vi "ULx Create 1D Waveform (1Samp).vi"(0 "t0":ext format="%#_10g", 5 "dt":dbl, 7 "data Array":dbl[](array[numeric]) format="%0.2f", 9 "channelName Array":string[](array[string]), 11 "error in":errorcluster) -> (4 "data":waveform(dbl)[](array[waveform]), 15 "error out":errorcluster)   [LabVIEW 2020]
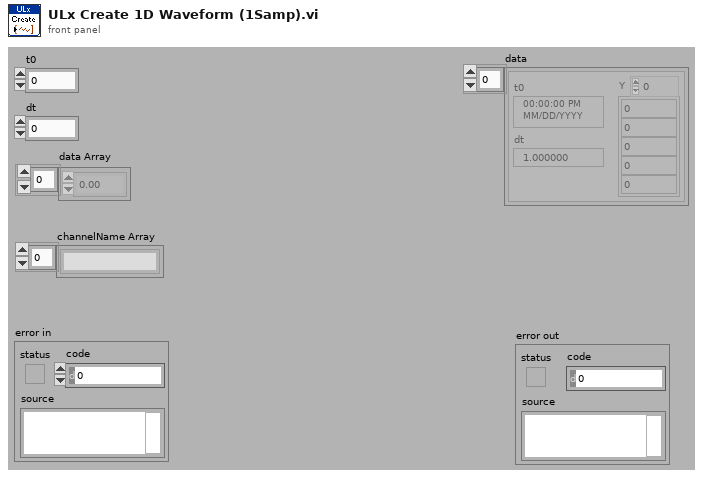
[diagram p1: front panel]
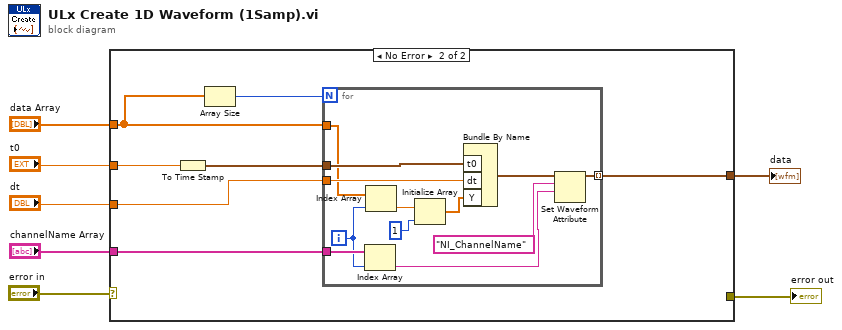
[diagram p0: block diagram]
diagram:
  n1 = case shown="No Error" "error in" {
    selector: "error in" -> [w8 _]
    tunnel: [w8 _] -> w6
    tunnel: "data Array" -> [_ w10]
    tunnel: "t0" -> [_ w14]
    tunnel: "dt" -> [_ w13]
    tunnel: "channelName Array" -> [_ w12]
    tunnel: [_ w11] -> w1
    frame Error {
    }
    frame No Error {
      n2 = To Time Stamp(1:w14) -> (0:w15:timestamp)
      n3 = Array Size(array=w10) -> (size(s)=w9:i32)
      n4 = for {
        N: w9 -> [_]
        tunnel: w10 -> [w20]
        tunnel: [w24] -> w11 mode=indexing
        tunnel: w15 -> [w27]
        tunnel: w13 -> [w26]
        tunnel: w12 -> [w21]
        i -> [w19]
        n5 = Index Array(array=w21, index=w19) -> (element=w22:string)
        n6 = Index Array(array=w20, index=w19) -> (element=w18:dbl)
        n7 = Initialize Array(w18, 1 ("dimension size")) -> (w16:dbl[])
        n8 = Bundle By Name("t0"=w27, "dt"=w26, "Y"=w16) -> (w25:waveform(dbl))  [unwired: 1 in]
        n9 = Set Waveform Attribute(5:w22, 6:"NI_ChannelName", 7:w25) -> (3:w24:waveform(dbl))  [unwired: 1 in, 2 out]
      }
    }
  }
  "error out" <- w6
  "data" <- w1
